vi "add_data_path.vi"(8 "error in (no error)":errorcluster, 11 "path_to_add":path) -> (0 "error out":errorcluster)   [LabVIEW 2015, in "lv-bin.lvlib" / "v1.lvlib"]
uses:
  v1.lvlib
  private/_controls/fg_command.ctl
  lv-bin.lvlib
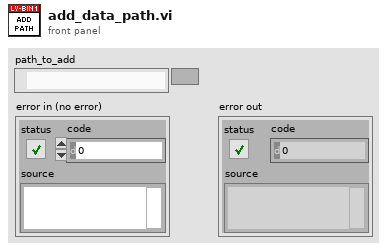
[diagram p1: front panel]
types:
  T1 = typedef "lv-bin.lvlib/fg_command.ctl" = enum16{"<fg_command>", "initialize", "read", "write", "shutdown", "<null>"}
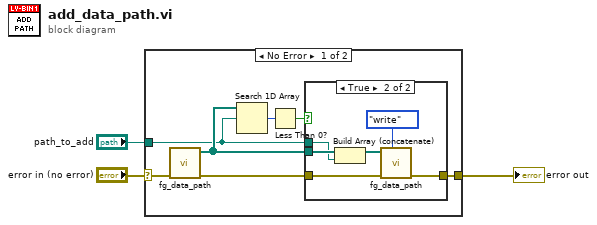
[diagram p0: block diagram]
diagram:
  n1 = case shown="No Error" "error in (no error)" {
    selector: "error in (no error)" -> [w4 w18]
    tunnel: "path_to_add" -> [w6 _]
    tunnel: [w5 w18] -> w1
    frame No Error {
      n2 = call "fg_data_path.vi"("error in (no error)"=w4) -> ("error out"=w10:errorcluster, "path [] out"=w9:path[])  [unwired: 9 in]
      n3 = Search 1D Array(1D array=w9, element=w6) -> (index of element=w8:i32)  [unwired: 1 in]
      n4 = Less Than 0?(x=w8) -> (x < 0?=w7:bool)
      n5 = case shown="True" w7 {
        tunnel: w10 -> [w11 w16]
        tunnel: w9 -> [_ w15]
        tunnel: w6 -> [_ w14]
        tunnel: [w11 w13] -> w5
        frame False {
        }
        frame True {
          n6 = Build Array (concatenate)(w15, w14) -> (w17:path[])
          n7 = call "fg_data_path.vi"("fg_command"=fg_command."write", "error in (no error)"=w16, "path [] in"=w17) -> ("error out"=w13:errorcluster)  [unwired: 7 in, 1 out]
        }
      }
    }
    frame Error {
    }
  }
  "error out" <- w1
